vi "SwissSPAD Live_Correct SS3 Gate Slippage [SGL].vi"(8 "Error In":errorcluster, 11 "Array in":sgl[][](array[numeric])) -> (0 "Error Out":errorcluster, 2 "Checkbox":bool, 3 "Array out":sgl[][](array[numeric]))   [LabVIEW 2021, in "SwissSPAD Live.lvlib"]
uses:
  SwissSPAD Live.lvlib
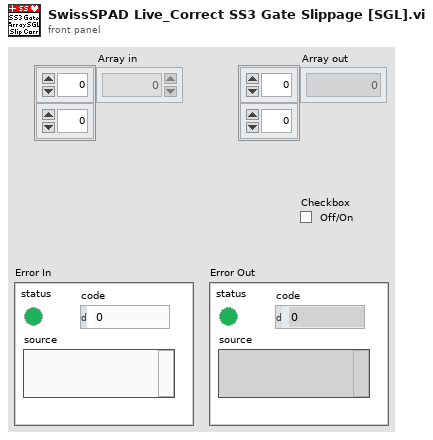
[diagram p1: front panel]
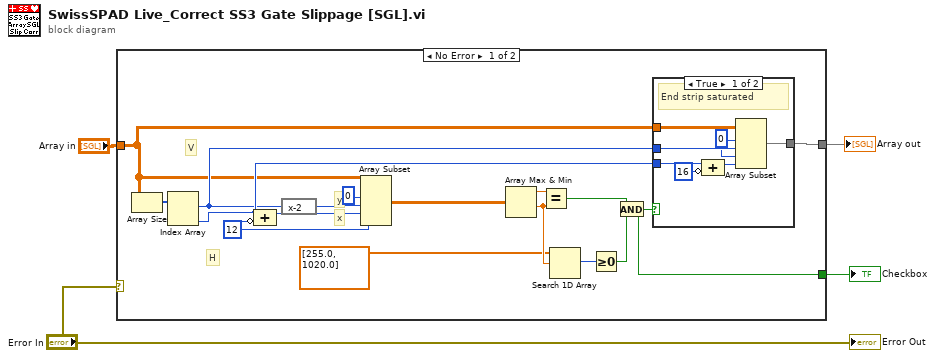
[diagram p0: block diagram]
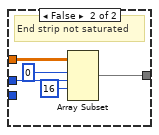
[diagram p2: hidden frame]
diagram:
  n1 = case shown="No Error" "Error In" {
    tunnel: [w17 _] -> w4
    tunnel: [w12 w34] -> w3
    tunnel: "Array in" -> [w11 w34]
    frame No Error {
      w10 = 12 ("value")
      # "H"
      # "V"
      # "x"
      # "y"
      n2 = Array Size(array=w11) -> (size(s)=w5:i32[])
      n3 = Index Array(array=w5) -> (element #1=w18:i32, element #2=w19:i32)  [unwired: 2 in]
      n4 = Compound Arithmetic op=ADD(w19, invert w10) -> (w9:i32)
      n5 = expression code="x-2"(w18) -> (w20:i32)
      n6 = Array Subset(array=w11, index (row)=0 ("length"), length (row)=w20, index (col)=w9, length (col)=w10) -> (w21:sgl[][])
      n7 = Array Max & Min(array=w21) -> (max value=w7:sgl, min value=w14:sgl)  [unwired: 2 out]
      n8 = Equal?(x=w7, y=w14) -> (x = y?=w8:bool)
      n9 = Search 1D Array(1D array=sgl[] [255.0, 1020.0] ("y"), element=w14) -> (index of element=w15:i32)  [unwired: 1 in]
      n10 = Greater Or Equal To 0?(x=w15) -> (x >= 0?=w16:bool)
      n11 = And(x=w8, y=w16) -> (x .and. y?=w17:bool)
      n12 = case shown="True" w17 {
        tunnel: w11 -> [w28 w33]
        tunnel: w18 -> [w27 w32]
        tunnel: [w25 w30] -> w12
        tunnel: w19 -> [w22 _]
        frame True {
          w26 = 0 ("index")
          # "End strip saturated"
          n13 = Compound Arithmetic op=ADD(w22, invert 16 ("value")) -> (w23:i32)
          n14 = Array Subset(array=w28, index (row)=w26, length (row)=w27, index (col)=w26, length (col)=w23) -> (w25:sgl[][])
        }
        frame False {
          # "End strip not saturated"
          n15 = Array Subset(array=w33, index (row)=0 ("index"), length (row)=w32, index (col)=16 ("index")) -> (w30:sgl[][])  [unwired: 1 in]
        }
      }
    }
    frame Error {
    }
  }
  "Checkbox" <- w4
  "Array out" <- w3
  "Error Out" <- "Error In"
